vi "GV gated pixelclock.vi"() -> ()   [LabVIEW 2017]
panel:
  out "GatedPixelclock":bool
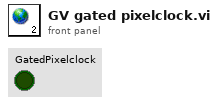
[diagram p1: front panel]
diagram:
